vi "Test_WriteValue_CheckDisk_ValuePresent.vi"(8 "error in (no error)":errorcluster, 11 "TestCase in":refnum<class "TestStreamToDiskTransport.lvclass">) -> (0 "error out":errorcluster, 3 "TestCase out":refnum<class "TestStreamToDiskTransport.lvclass">)   [LabVIEW 2017, in "TestStreamToDiskTransport.lvclass"]
uses:
  TestStreamToDiskTransport.lvclass
  TestStreamToDiskTransport.lvclass/TestStreamToDiskTransport.ctl
  Source/Concrete/StreamToDiskTransport/StreamToDiskTransport.lvclass/StreamToDiskTransport.ctl
  <vilib>/Utility/error.llb/Clear Errors.vi
  Source/Concrete/StreamToDiskTransport/StreamToDiskTransport.lvclass
  C:/Git/composed-transport/Source/ITransport/ITransport.lvclass
  Source/ITransport/ITransport.lvclass
panel:
  out "Test File Path":path
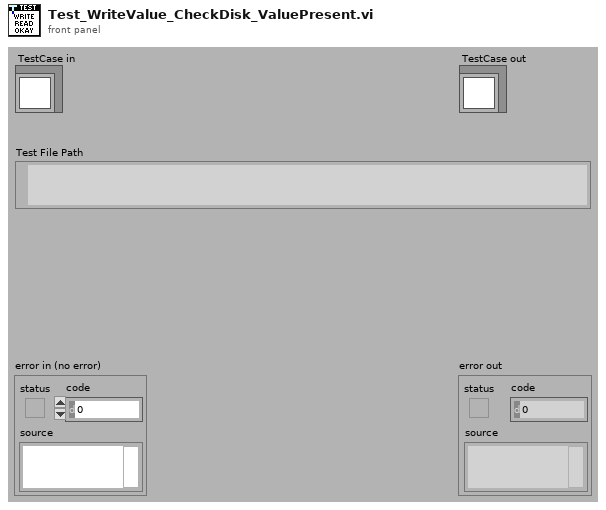
[diagram p1: front panel]
types:
  T1 = enum16{"open", "open or create", "create or replace", "create", "open (read-only)"}
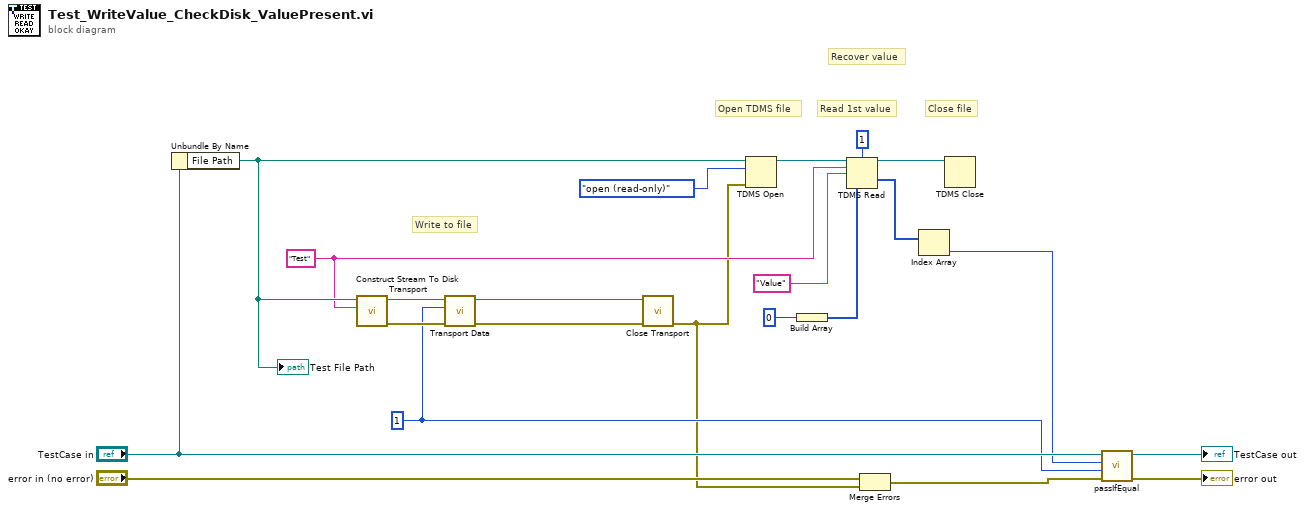
[diagram p0: block diagram]
diagram:
  w5 = "Test" ("Key Name")
  w4 = 1 ("Test Value")
  # "Close file"
  # "Open TDMS file"
  # "Read 1st value"
  # "Recover value"
  # "Write to file"
  n1 = Unbundle By Name("TestCase in") -> ("File Path"=w6:path)
  "Test File Path" <- w6
  n2 = call "Construct Stream To Disk Transport.vi"("Channel Name"=w5, "File Path"=w6) -> ("error out"=w22:errorcluster, "StreamToDiskTransport"=w17:refnum<class "StreamToDiskTransport.lvclass">)  [unwired: 8 in]
  n3 = call "Transport Data.vi"("error in (no error)"=w22, "Value"=w4, "ITransport in"=w17) -> ("error out"=w16:errorcluster, "ITransport out"=w1:refnum<class "StreamToDiskTransport.lvclass">)  [unwired: 7 in]
  n4 = call-dynamic "Close Transport.vi"("error in (no error)"=w16, "StreamToDiskTransport"=w1) -> ("error out"=w2:errorcluster)  [unwired: 9 in]
  n5 = TDMS Open(8:w2, 10:T1."open (read-only)" ("operation (0:open)"), 11:w6) -> (3:w14:refnum<k34>)  [unwired: 4 in, 1 out]
  n6 = Build Array(0) -> (w10:i32[])
  n7 = TDMS Read(0:w14, 2:i64 1 ("count (-1: all)"), 5:w5, 7:"Value" ("channel name(s) in"), 12:w10) -> (4:w9:refnum<k34>, 10:w8:i32[])  [unwired: 3 in, 4 out]
  n8 = Merge Errors("error in (no error)", w2) -> (w18:errorcluster)
  n9 = Index Array(array=w8) -> (element=w3:i32)  [unwired: 1 in]
  n10 = TDMS Close(11:w9) -> ()  [unwired: 1 in, 2 out]
  n11 = call-dynamic "passIfEqual.vi"("error in (no error)"=w18, "y"=w4, "x"=w3, "TestCase in"="TestCase in") -> ("error out"=→"error out":errorcluster, "TestCase out"=→"TestCase out":refnum<class "TestStreamToDiskTransport.lvclass">)  [unwired: 6 in]
